vi "Read Freezer.vi"(11 "Heater in":refnum<class "Heater.lvclass">) -> (2 "Freezer":T1, 3 "Heater out":refnum<class "Heater.lvclass">)   [LabVIEW 2015, in "cRIO-Carbondioxide.lvlib" / "CO2-Actor.lvlib" / "Heater.lvclass"]
uses:
  Heater.lvclass
  cRIO-CO2/Freezers Enumerator.ctl
  Heater.lvclass/Heater.ctl
  cRIO-CO2/cRIO-CO2.lvclass
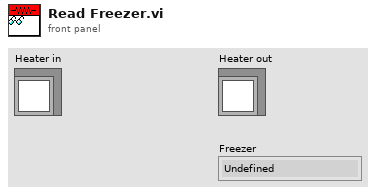
[diagram p1: front panel]
types:
  T1 = typedef "cRIO-Carbondioxide.lvlib/cRIO-CO2.lvlib/cRIO-CO2.lvclass/Freezers Enumerator.ctl" = enum16{"Undefined", "Syringe", "Cold Tank 1", "Cold Tank 2", "Cold Tank 3", "Cold Tank 4"}
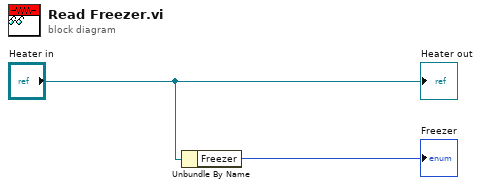
[diagram p0: block diagram]
diagram:
  n1 = Unbundle By Name("Heater in") -> ("Freezer"=→"Freezer":T1)
  "Heater out" <- "Heater in"
